vi "LEP_RV_GetTCPDefaultIP.vi"() -> (0 "IP address":string[](array[string]))   [LabVIEW 2011]
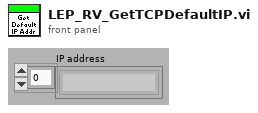
[diagram p1: front panel]
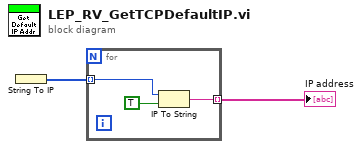
[diagram p0: block diagram]
diagram:
  n1 = String To IP() -> (0:w1:u32[])  [unwired: 1 in]
  n2 = for {
    tunnel: [w5] -> w2 mode=indexing
    tunnel: w1 -> [w3] mode=indexing
    n3 = IP To String(1:TRUE ("dot notation? (F)"), 2:w3) -> (0:w5:string)
  }
  "IP address" <- w2
